vi "CaliperResultToString.vi"(9 "Result":T1, 11 "CaliperType_w_Pic":T2 caption="Caliper Type" items=["Distance", "Mid Point", "Perpendicular Projection", "Lines Intersection", "Angle from Horizontal", "Angle from Vertical", "Angle Defined by 3 Points", "Angle Defined by 4 Points", "Bissecting Line", "Mid Line", "Center of Mass", "Area", "Line Fit", "Circle Fit", "Ellipse Fit"]) -> (3 "ResultString":string)   [LabVIEW 2019]
uses:
  Controls/CaliperType with Picture.ctl
  Controls/CaliperResult.ctl
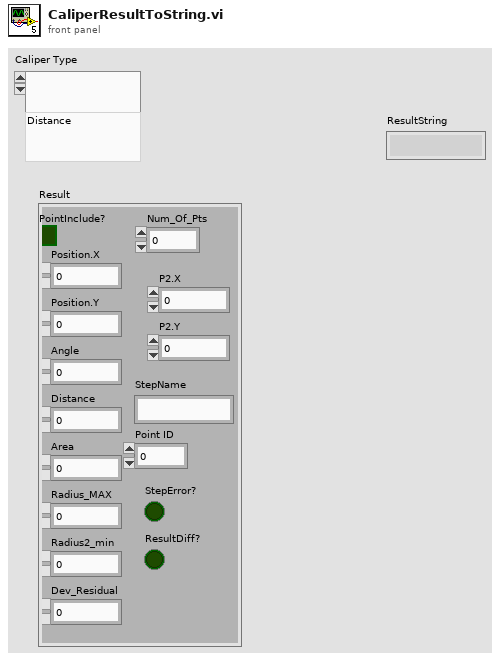
[diagram p1: front panel]
types:
  T1 = typedef "CaliperResult.ctl" = cluster{"PointInclude?":bool, "Num_Of_Pts":u8, "Position.X":dbl, "Position.Y":dbl, "Angle":dbl, "Distance":dbl, "Area":dbl, "Radius_MAX":dbl, "Radius2_min":dbl, "Dev_Residual":dbl, "P2.X":dbl, "P2.Y":dbl, "StepName":string, "Point ID":u8, "StepError?":bool, "ResultDiff?":bool}
  T2 = typedef "CaliperType with Picture.ctl" = u32
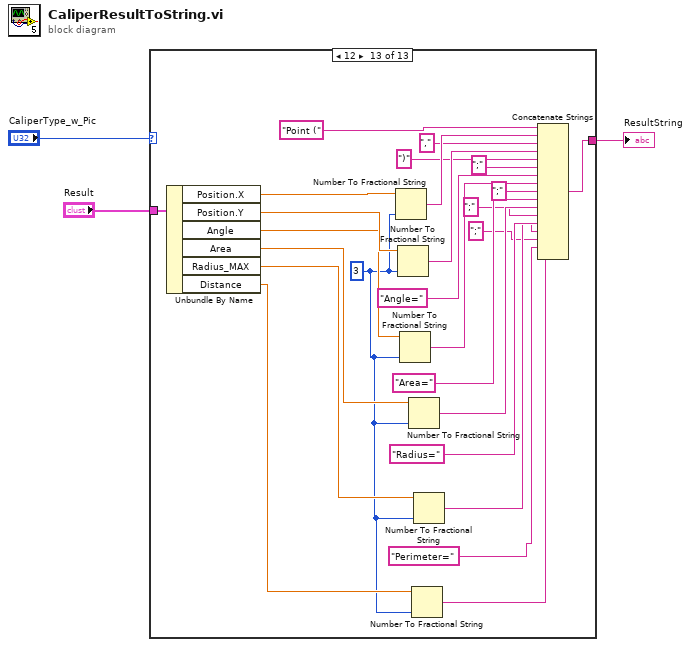
[diagram p0: block diagram]
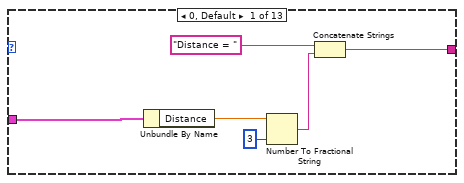
[diagram p2: hidden frame]
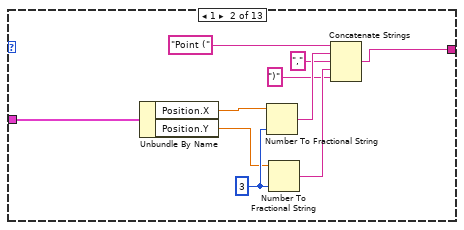
[diagram p3: hidden frame]
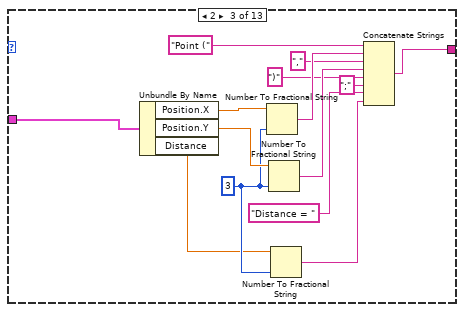
[diagram p4: hidden frame]
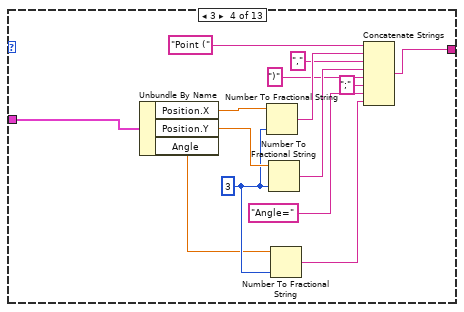
[diagram p5: hidden frame]
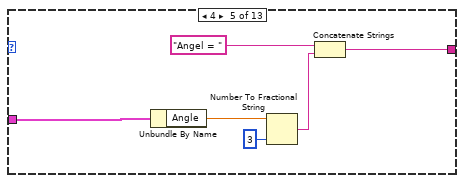
[diagram p6: hidden frame]
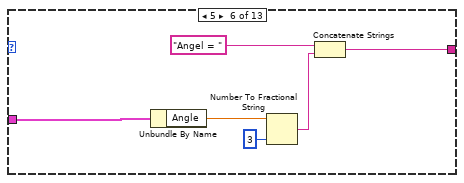
[diagram p7: hidden frame]
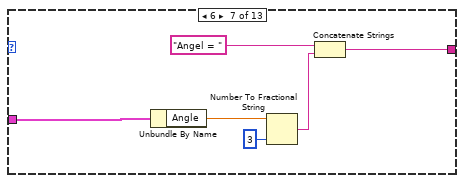
[diagram p8: hidden frame]
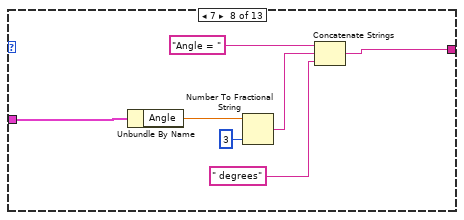
[diagram p9: hidden frame]
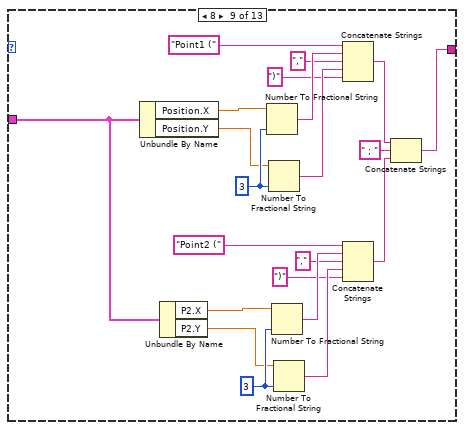
[diagram p10: hidden frame]
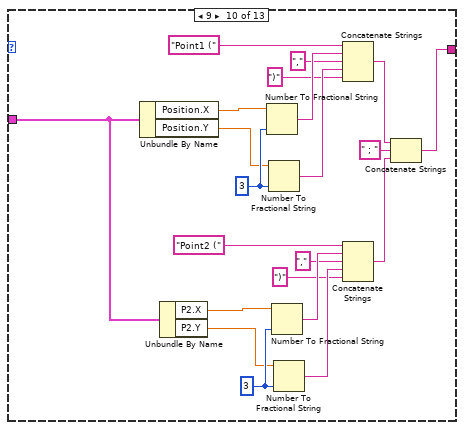
[diagram p11: hidden frame]
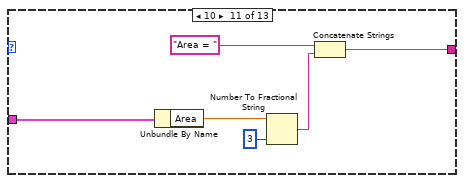
[diagram p12: hidden frame]
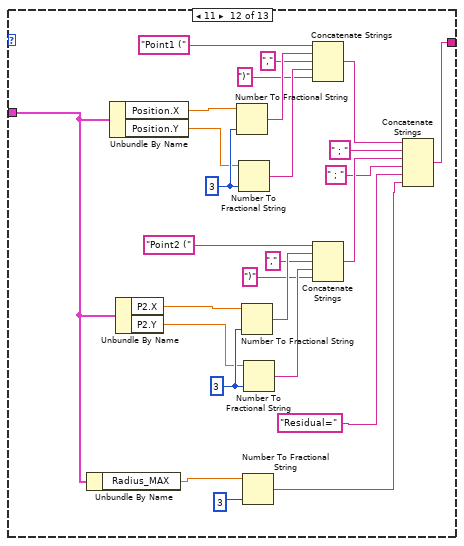
[diagram p13: hidden frame]
diagram:
  n1 = case shown="12" "CaliperType_w_Pic" {
    tunnel: "Result" -> [w9 w19 w33 w47 w53 w59 w65 w72 w77 w98 w120 w125 w163]
    tunnel: [w4 w16 w30 w44 w48 w54 w60 w67 w73 w94 w115 w127 w149] -> w1
    frame 0, Default {
      n2 = Unbundle By Name(w9) -> ("Distance"=w8:dbl)
      n3 = Number To Fractional String(number=w8, precision (6)=i16 3) -> (F-format string=w5:string)  [unwired: 2 in]
      n4 = Concatenate Strings("Distance = ", w5) -> (w4:string)
    }
    frame 1 {
      w15 = i16 3 ("precision (6)")
      n5 = Unbundle By Name(w19) -> ("Position.X"=w18:dbl, "Position.Y"=w14:dbl)
      n6 = Number To Fractional String(number=w18, precision (6)=w15) -> (F-format string=w13:string)  [unwired: 2 in]
      n7 = Number To Fractional String(number=w14, precision (6)=w15) -> (F-format string=w11:string)  [unwired: 2 in]
      n8 = Concatenate Strings("Point (", w13, "," ("string"), w11, ")" ("string")) -> (w16:string)
    }
    frame 2 {
      w24 = i16 3 ("precision (6)")
      n9 = Unbundle By Name(w33) -> ("Position.X"=w32:dbl, "Position.Y"=w29:dbl, "Distance"=w23:dbl)
      n10 = Number To Fractional String(number=w32, precision (6)=w24) -> (F-format string=w28:string)  [unwired: 2 in]
      n11 = Number To Fractional String(number=w29, precision (6)=w24) -> (F-format string=w26:string)  [unwired: 2 in]
      n12 = Number To Fractional String(number=w23, precision (6)=w24) -> (F-format string=w20:string)  [unwired: 2 in]
      n13 = Concatenate Strings("Point (", w28, "," ("string"), w26, ")" ("string"), ";" ("string"), "Distance = ", w20) -> (w30:string)
    }
    frame 3 {
      w38 = i16 3 ("precision (6)")
      n14 = Unbundle By Name(w47) -> ("Position.X"=w46:dbl, "Position.Y"=w43:dbl, "Angle"=w37:dbl)
      n15 = Number To Fractional String(number=w46, precision (6)=w38) -> (F-format string=w42:string)  [unwired: 2 in]
      n16 = Number To Fractional String(number=w43, precision (6)=w38) -> (F-format string=w40:string)  [unwired: 2 in]
      n17 = Number To Fractional String(number=w37, precision (6)=w38) -> (F-format string=w34:string)  [unwired: 2 in]
      n18 = Concatenate Strings("Point (", w42, "," ("string"), w40, ")" ("string"), ";" ("string"), "Angle=", w34) -> (w44:string)
    }
    frame 4 {
      n19 = Unbundle By Name(w53) -> ("Angle"=w52:dbl)
      n20 = Number To Fractional String(number=w52, precision (6)=i16 3) -> (F-format string=w49:string)  [unwired: 2 in]
      n21 = Concatenate Strings("Angel = ", w49) -> (w48:string)
    }
    frame 5 {
      n22 = Unbundle By Name(w59) -> ("Angle"=w58:dbl)
      n23 = Number To Fractional String(number=w58, precision (6)=i16 3) -> (F-format string=w55:string)  [unwired: 2 in]
      n24 = Concatenate Strings("Angel = ", w55) -> (w54:string)
    }
    frame 6 {
      n25 = Unbundle By Name(w65) -> ("Angle"=w64:dbl)
      n26 = Number To Fractional String(number=w64, precision (6)=i16 3) -> (F-format string=w61:string)  [unwired: 2 in]
      n27 = Concatenate Strings("Angel = ", w61) -> (w60:string)
    }
    frame 7 {
      n28 = Unbundle By Name(w72) -> ("Angle"=w71:dbl)
      n29 = Number To Fractional String(number=w71, precision (6)=i16 3) -> (F-format string=w68:string)  [unwired: 2 in]
      n30 = Concatenate Strings("Angle = ", w68, " degrees") -> (w67:string)
    }
    frame 8 {
      w83 = i16 3 ("precision (6)")
      w91 = i16 3 ("precision (6)")
      n31 = Unbundle By Name(w77) -> ("Position.X"=w93:dbl, "Position.Y"=w90:dbl)
      n32 = Unbundle By Name(w77) -> ("P2.X"=w85:dbl, "P2.Y"=w82:dbl)
      n33 = Number To Fractional String(number=w93, precision (6)=w91) -> (F-format string=w89:string)  [unwired: 2 in]
      n34 = Number To Fractional String(number=w90, precision (6)=w91) -> (F-format string=w87:string)  [unwired: 2 in]
      n35 = Number To Fractional String(number=w85, precision (6)=w83) -> (F-format string=w81:string)  [unwired: 2 in]
      n36 = Number To Fractional String(number=w82, precision (6)=w83) -> (F-format string=w79:string)  [unwired: 2 in]
      n37 = Concatenate Strings("Point1 (", w89, "," ("string"), w87, ")" ("string")) -> (w75:string)
      n38 = Concatenate Strings("Point2 (", w81, "," ("string"), w79, ")" ("string")) -> (w74:string)
      n39 = Concatenate Strings(w75, " ; " ("string"), w74) -> (w73:string)
    }
    frame 9 {
      w104 = i16 3 ("precision (6)")
      w112 = i16 3 ("precision (6)")
      n40 = Unbundle By Name(w98) -> ("Position.X"=w114:dbl, "Position.Y"=w111:dbl)
      n41 = Unbundle By Name(w98) -> ("P2.X"=w106:dbl, "P2.Y"=w103:dbl)
      n42 = Number To Fractional String(number=w114, precision (6)=w112) -> (F-format string=w110:string)  [unwired: 2 in]
      n43 = Number To Fractional String(number=w111, precision (6)=w112) -> (F-format string=w108:string)  [unwired: 2 in]
      n44 = Number To Fractional String(number=w106, precision (6)=w104) -> (F-format string=w102:string)  [unwired: 2 in]
      n45 = Number To Fractional String(number=w103, precision (6)=w104) -> (F-format string=w100:string)  [unwired: 2 in]
      n46 = Concatenate Strings("Point1 (", w110, "," ("string"), w108, ")" ("string")) -> (w96:string)
      n47 = Concatenate Strings("Point2 (", w102, "," ("string"), w100, ")" ("string")) -> (w95:string)
      n48 = Concatenate Strings(w96, " ; " ("string"), w95) -> (w94:string)
    }
    frame 10 {
      n49 = Unbundle By Name(w120) -> ("Area"=w119:dbl)
      n50 = Number To Fractional String(number=w119, precision (6)=i16 3) -> (F-format string=w116:string)  [unwired: 2 in]
      n51 = Concatenate Strings("Area = ", w116) -> (w115:string)
    }
    frame 11 {
      w136 = i16 3 ("precision (6)")
      w144 = i16 3 ("precision (6)")
      n52 = Unbundle By Name(w125) -> ("Radius_MAX"=w124:dbl)
      n53 = Unbundle By Name(w125) -> ("Position.X"=w146:dbl, "Position.Y"=w143:dbl)
      n54 = Unbundle By Name(w125) -> ("P2.X"=w138:dbl, "P2.Y"=w135:dbl)
      n55 = Number To Fractional String(number=w146, precision (6)=w144) -> (F-format string=w142:string)  [unwired: 2 in]
      n56 = Number To Fractional String(number=w143, precision (6)=w144) -> (F-format string=w140:string)  [unwired: 2 in]
      n57 = Number To Fractional String(number=w138, precision (6)=w136) -> (F-format string=w134:string)  [unwired: 2 in]
      n58 = Number To Fractional String(number=w124, precision (6)=i16 3) -> (F-format string=w121:string)  [unwired: 2 in]
      n59 = Number To Fractional String(number=w135, precision (6)=w136) -> (F-format string=w132:string)  [unwired: 2 in]
      n60 = Concatenate Strings("Point1 (", w142, "," ("string"), w140, ")" ("string")) -> (w129:string)
      n61 = Concatenate Strings("Point2 (", w134, "," ("string"), w132, ")" ("string")) -> (w128:string)
      n62 = Concatenate Strings(w129, " ; " ("string"), w128, " ; " ("string"), "Residual=", w121) -> (w127:string)
    }
    frame 12 {
      w156 = i16 3 ("precision (6)")
      n63 = Unbundle By Name(w163) -> ("Position.X"=w172:dbl, "Position.Y"=w170:dbl, "Angle"=w165:dbl, "Area"=w160:dbl, "Radius_MAX"=w158:dbl, "Distance"=w157:dbl)
      n64 = Number To Fractional String(number=w172, precision (6)=w156) -> (F-format string=w169:string)  [unwired: 2 in]
      n65 = Number To Fractional String(number=w170, precision (6)=w156) -> (F-format string=w167:string)  [unwired: 2 in]
      n66 = Number To Fractional String(number=w165, precision (6)=w156) -> (F-format string=w164:string)  [unwired: 2 in]
      n67 = Number To Fractional String(number=w160, precision (6)=w156) -> (F-format string=w159:string)  [unwired: 2 in]
      n68 = Number To Fractional String(number=w157, precision (6)=w156) -> (F-format string=w150:string)  [unwired: 2 in]
      n69 = Number To Fractional String(number=w158, precision (6)=w156) -> (F-format string=w153:string)  [unwired: 2 in]
      n70 = Concatenate Strings("Point (", w169, "," ("string"), w167, ")" ("string"), ";" ("string"), "Angle=", w164, ";" ("string"), "Area=", w159, ";" ("string"), "Radius=", w153, ";" ("string"), "Perimeter=", w150) -> (w149:string)
    }
  }
  "ResultString" <- w1
